vi "read Port.vi"(8 "error in (no error)":errorcluster, 9 "length":i32, 10 "packet":string, 11 "port_num":i32) -> (0 "error out":errorcluster, 2 "packet out":string, 3 "function return":i32)   [LabVIEW 2018, in "labview.lvlib"]
doc: "WINDECLSPEC int readPort (int port_num, uint8_t *packet, int length);"
uses:
  labview.lvlib
  dxl_x86_c.dll
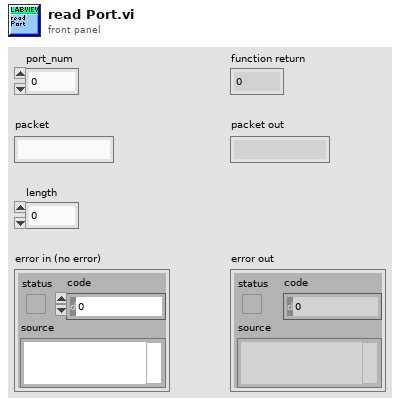
[diagram p1: front panel]
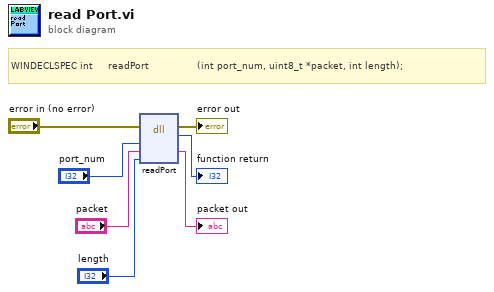
[diagram p0: block diagram]
diagram:
  # "WINDECLSPEC int     readPort                (int port_num, uint8_t *packet, int length);"
  n1 = dll-call lib="C:/Users/joaos/OneDrive/Documents/[PhD]/Project Omnidirectional Vehicle/Vanes/LabView_code/joaoandthethreestands/DynamixelSDK-3.7.31/labview/new_compilation/dxl_x86_c.*" fn="readPort"(error in="error in (no error)", "port_num"="port_num", "packet"="packet", "length"="length") -> (error out=→"error out":errorcluster, →"function return":i32, "packet"=→"packet out":string)  [unwired: 4 in, 1 out]
